vi "main.vi"(8 "error in":errorcluster) -> (0 "error out":errorcluster)   [LabVIEW 2018, in "Wash Display Console.lvlib"]
uses:
  Wash Display Console.lvlib
  Common/Common.lvlib
  Common/vi/Stop All - Action.ctl
  ctl/Queue Actions.ctl
  ctl/Module State.ctl
  Error Handler/Error Handler/ctl/Module State.ctl
  Error Handler/Error Handler/Error Handler.lvlib
  Controller/Controller.lvlib
  Controller/ctl/Module State.ctl
  ctl/Car Wash Indicators.ctl
  Common/ctl/Wash Step.ctl
  ctl/Wash Entry.ctl
  ctl/Vehicle Out of Position.ctl
panel:
  out "Car Wash Indicators":T1
  out "Time Remaining":dbl format="%07.2g"
  out "Vehicle Out of Position?":T2
  out "Wash Entry":T3
  # "Wash Display Console"
  # "[Covers: UI1]"
  # "[Covers: UI3]"
  # "[Covers: UI3A1]\n[Covers: UI3A2]\n[Covers: UI3A3]"
  # "[Covers: UI3B]\n[Covers: UI3B1]"
  # "true = red"
  # "[Covers: UI3D]\n[Covers: UI3D1]"
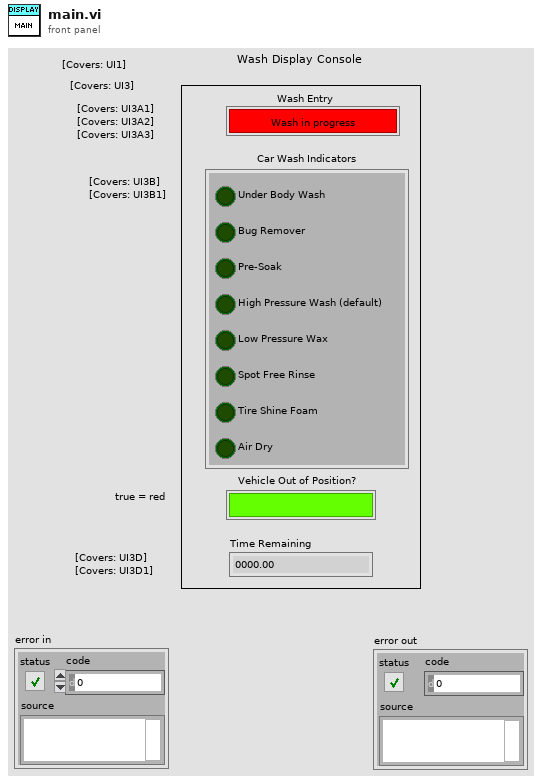
[diagram p1: front panel]
types:
  T1 = typedef "Wash Display Console.lvlib/Car Wash Indicators.ctl" = cluster{"Under Body Wash":bool, "Bug Remover":bool, "Pre-Soak":bool, "High Pressure Wash (default)":bool, "Low Pressure Wax":bool, "Spot Free Rinse":bool, "Tire Shine Foam":bool, "Air Dry":bool}
  T2 = typedef "Wash Display Console.lvlib/Vehicle Out of Position.ctl" = bool
  T3 = typedef "Wash Display Console.lvlib/Wash Entry.ctl" = bool
  T4 = typedef "Wash Display Console.lvlib/Module State.ctl" = enum16{"Init", "Idle", "Error", "Close", "Car Wash Indicators: Set All", "Car Wash Indicators: Set Single (On/Off)", "Wash Entry: Set State", "Vehicle Out of Position: Green/Red", "Time Remaining: Set"}
  T5 = typedef "Wash Display Console.lvlib/Queue Actions.ctl" = enum16{"Create", "Get", "Destroy"}
  T6 = typedef "Common.lvlib/Stop All - Action.ctl" = enum16{"Create", "Get", "Fire", "Destroy"}
  T7 = typedef "Controller.lvlib/Module State.ctl" = enum16{"Init", "Idle", "Error", "Close", "Wait for Start State", "Start State", "Wait For Vehicle Position", "Wash Step Execution", "Wash Step/Cycle Completion", "Wash Exit State", "Wash Abort/Terminate State", "Entry Console: Start button pressed", "Entry Console: Wash Steps buttons Pressed", "Vehicle Position: Slider Moved", "Check Timer"}
  T8 = typedef "Error Handler.lvlib/Module State.ctl" = enum16{"Init", "Idle", "Error", "Close", "Handle External Error", "Log Error"}
  T9 = typedef "Common.lvlib/Wash Step.ctl" = enum16{"None", "Under Body Wash", "Bug Remover", "Pre-Soak", "High Pressure Wash (default)", "Low Pressure Wax", "Spot Free Rinse", "Tire Shine Foam", "Air Dry"}
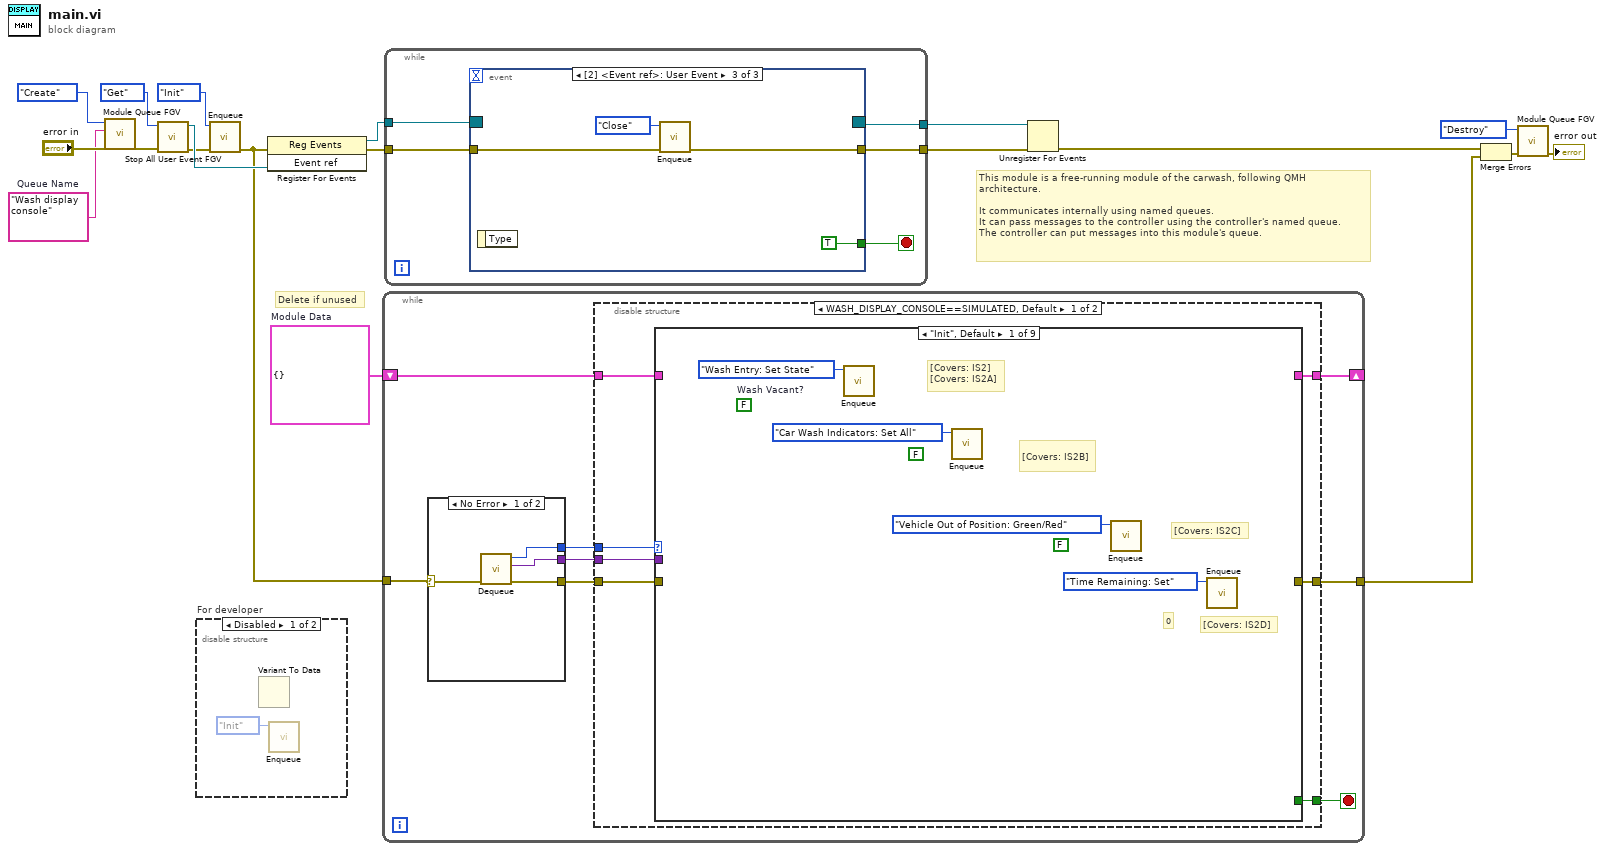
[diagram p0: block diagram]
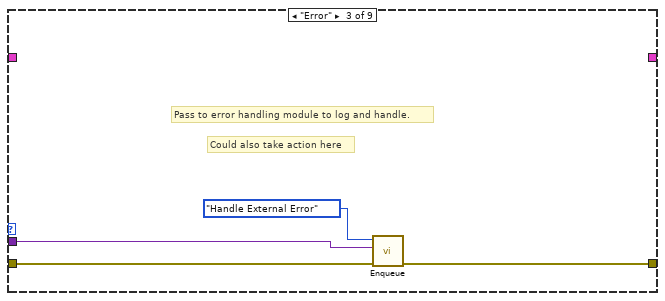
[diagram p4: hidden frame]
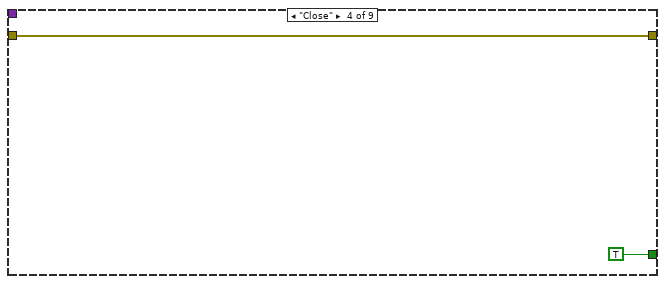
[diagram p5: hidden frame]
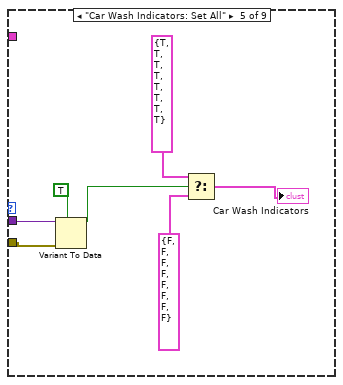
[diagram p6: hidden frame]
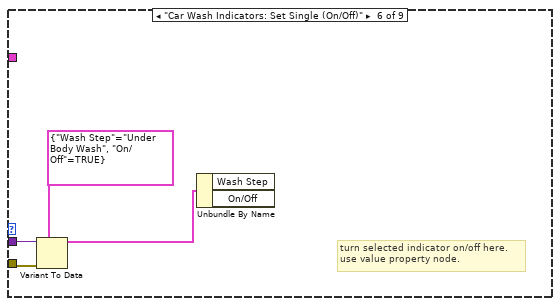
[diagram p7: hidden frame]
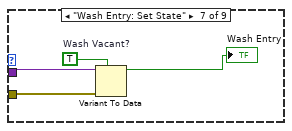
[diagram p8: hidden frame]
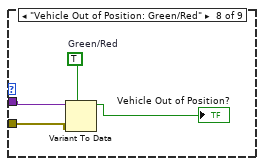
[diagram p9: hidden frame]
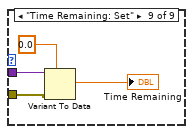
[diagram p10: hidden frame]
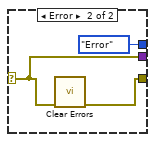
[diagram p12: hidden frame]
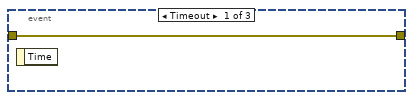
[diagram p13: hidden frame]
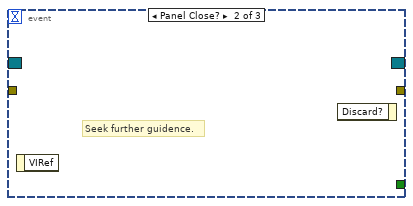
[diagram p14: hidden frame]
diagram:
  w1 = "Wash display console"  # Queue Name
  w6 = cluster{} {}  # Module Data
  # "This module is a free-running module of the carwash, following QMH\narchitecture.\n\nIt communicates internally using named queues.\nIt can pass messages to the controller using the controller's named queue.\nThe controller can put messages into this module's queue."
  # "Delete if unused"
  n1 = call "Module Queue FGV.vi"("error in"="error in", "Queue Name"=w1, "Action"=Queue_Actions."Create") -> ("error out"=w16:errorcluster)  [unwired: 7 in, 1 out]
  n2 = call "Stop All User Event FGV.vi"("error in"=w16, "Action"=Stop_All_-_Action."Get") -> ("error out"=w15:errorcluster, "Event ref"=w18:refnum<user-event>)  [unwired: 8 in]
  n3 = disable-structure "For developer" shown="Disabled" {
    frame Disabled {
      n4 = Variant To Data() -> ()  [unwired: 3 in, 2 out]
      n5 = call "Enqueue.vi"("State"=Module_State."Init") -> ()  [unwired: 10 in, 1 out]
    }
    frame Enabled {
    }
  }
  n6 = call "Enqueue.vi"("error in"=w15, "State"=Module_State."Init") -> ("error out"=w7:errorcluster)  [unwired: 9 in]
  n7 = register-events(error in=w7, w18) -> (reference out=w13:refnum<event-registration>, error out=w11:errorcluster)  [unwired: 1 in]
  n8 = while {
    tunnel: w7 -> [w28]
    shift-right: [w23] -> _
    shift-left: w6 -> [w24]
    tunnel: [w21] -> w5
    stop <- w22 stop-if-true
    n9 = case shown="No Error" w28 {
      selector: w28 -> [w73 w75]
      tunnel: [w72 w76] -> w25
      tunnel: [w71 w75] -> w26
      tunnel: [w70 Module_State."Error" ("State")] -> w27
      frame No Error {
        n10 = call "Dequeue.vi"("error in"=w73) -> ("error out"=w72:errorcluster, "Data"=w71:variant, "State"=w70:T4)  [unwired: 8 in]
      }
      frame Error {
        n11 = call <vilib>:"Clear Errors.vi"("error in (no error)"=w75) -> ("error out"=w76:errorcluster)  [unwired: 5 in, 1 out]
      }
    }
    n12 = disable-structure shown="WASH_DISPLAY_CONSOLE==SIMULATED, Default" {
      disable-tunnel: w27 -> [w35 _]
      disable-tunnel: w26 -> [w34 _]
      disable-tunnel: w25 -> [w33 _]
      disable-tunnel: w24 -> [w32 _]
      disable-tunnel: [w31 _] -> w23
      disable-tunnel: [w30 _] -> w22
      disable-tunnel: [w29 _] -> w21
      frame condition #0 (active) {
        n13 = case shown="\"Init\", Default" w35 {
          tunnel: w34 -> [_ _ w42 _ w53 w55 w60 w65 w68]
          tunnel: w33 -> [_ _ w41 w45 w51 w57 w58 w64 w67]
          tunnel: w32 -> [_ w40 _ _ _ _ _ _ _]
          tunnel: [_ w40 _ _ _ _ _ _ _] -> w31
          tunnel: [_ _ _ TRUE _ _ _ _ _] -> w30
          tunnel: [_ _ w43 w45 _ _ _ _ _] -> w29
          frame "Init", Default {
            (unwired) T3 FALSE  # Wash Vacant?
            (unwired) FALSE
            (unwired) FALSE
            # "[Covers: IS2D]"
            # "[Covers: IS2C]"
            # "[Covers: IS2B]"
            # "[Covers: IS2]\n[Covers: IS2A]"
            # "0"
            n14 = call "Enqueue.vi"("State"=Module_State."Wash Entry: Set State") -> ()  [unwired: 10 in, 1 out]
            n15 = call "Enqueue.vi"("State"=Module_State."Car Wash Indicators: Set All") -> ()  [unwired: 10 in, 1 out]
            n16 = call "Enqueue.vi"("State"=Module_State."Vehicle Out of Position: Green/Red") -> ()  [unwired: 10 in, 1 out]
            n17 = call "Enqueue.vi"("State"=Module_State."Time Remaining: Set") -> ()  [unwired: 10 in, 1 out]
          }
          frame "Idle" {
          }
          frame "Error" {
            # "Could also take action here"
            # "Pass to error handling module to log and handle."
            n18 = call "Enqueue.vi"("error in"=w41, "Data"=w42, "State"=Module_State."Handle External Error") -> ("error out"=w43:errorcluster)  [unwired: 8 in]
          }
          frame "Close" {
          }
          frame "Car Wash Indicators: Set All" {
            n19 = Variant To Data(error in=w51, type=TRUE, Variant=w53) -> (data=w47:bool)  [unwired: 1 out]
            n20 = Select(t=T1 {"Under Body Wash"=TRUE, "Bug Remover"=TRUE, "Pre-Soak"=TRUE, "High Pressure Wash (default)"=TRUE, "Low Pressure Wax"=TRUE, "Spot Free Rinse"=TRUE, "Tire Shine Foam"=TRUE, "Air Dry"=TRUE} ("Car Wash Indicators"), s=w47, f=T1 {"Under Body Wash"=FALSE, "Bug Remover"=FALSE, "Pre-Soak"=FALSE, "High Pressure Wash (default)"=FALSE, "Low Pressure Wax"=FALSE, "Spot Free Rinse"=FALSE, "Tire Shine Foam"=FALSE, "Air Dry"=FALSE} ("Car Wash Indicators")) -> (s? t:f=→"Car Wash Indicators":T1)
          }
          frame "Car Wash Indicators: Set Single (On/Off)" {
            # "turn selected indicator on/off here.\nuse value property node."
            n21 = Variant To Data(error in=w57, type=cluster{"Wash Step":T9, "On/Off":bool} {"Wash Step"=enum."Under Body Wash", "On/Off"=TRUE}, Variant=w55) -> (data=w54:cluster{"Wash Step":T9, "On/Off":bool})  [unwired: 1 out]
            n22 = Unbundle By Name(w54) -> ()  [unwired: 2 out]
          }
          frame "Wash Entry: Set State" {
            w61 = TRUE  # Wash Vacant?
            n23 = Variant To Data(error in=w58, type=w61, Variant=w60) -> (data=→"Wash Entry":bool)  [unwired: 1 out]
          }
          frame "Vehicle Out of Position: Green/Red" {
            w63 = TRUE  # Green/Red
            n24 = Variant To Data(error in=w64, type=w63, Variant=w65) -> (data=→"Vehicle Out of Position?":bool)  [unwired: 1 out]
          }
          frame "Time Remaining: Set" {
            n25 = Variant To Data(error in=w67, type=0.0, Variant=w68) -> (data=→"Time Remaining":dbl)  [unwired: 1 out]
          }
        }
      }
      frame condition #1 {
        # "Write hardware code here"
      }
    }
  }
  n26 = while {
    tunnel: w13 -> [w81]
    tunnel: [w80] -> w12
    tunnel: [w79] -> w10
    tunnel: w11 -> [w78]
    stop <- w77 stop-if-true
    n27 = event shown="[2] <Event ref>: User Event" {
      selector: w81 -> [_ _ _]
      dyn-events: [_ _ _] -> w80
      timeout: _ -> [_ _ _]
      tunnel: [w82 _ w85] -> w79
      tunnel: w78 -> [w82 _ w86]
      tunnel: [_ _ TRUE] -> w77
      event Timeout {
        n28 = event-data() -> ()  [unwired: 1 in, 1 out]
      }
      event Panel Close? {
        # "Seek further guidence."
        n29 = event-data() -> ()  [unwired: 1 in, 1 out]
        n30 = event-data() -> ()  [unwired: 2 in, 1 out]
      }
      event User Event {
        n31 = event-data() -> ()  [unwired: 1 in, 1 out]
        n32 = call "Enqueue.vi"("error in"=w86, "State"=Module_State."Close") -> ("error out"=w85:errorcluster)  [unwired: 9 in]
      }
    }
  }
  n33 = Unregister For Events(event registration refnum=w12, error in=w10) -> (error out=w2:errorcluster)
  n34 = Merge Errors(w2, w5) -> (w4:errorcluster)
  n35 = call "Module Queue FGV.vi"("error in"=w4, "Action"=Queue_Actions."Destroy") -> ("error out"=→"error out":errorcluster)  [unwired: 8 in, 1 out]
